vi "Send Barcode.vi"(8 "ErrorIn":errorcluster, 10 "Command":string, 11 "VISAIn":refnum<visa-resource-name>) -> (0 "ErrorOut":errorcluster, 2 "Data":string, 3 "VISAOut":refnum<visa-resource-name>)   [LabVIEW 2017, in "I28Drivers.lvlib"]
uses:
  I28Drivers.lvlib
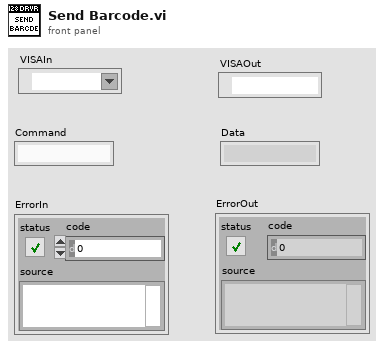
[diagram p1: front panel]
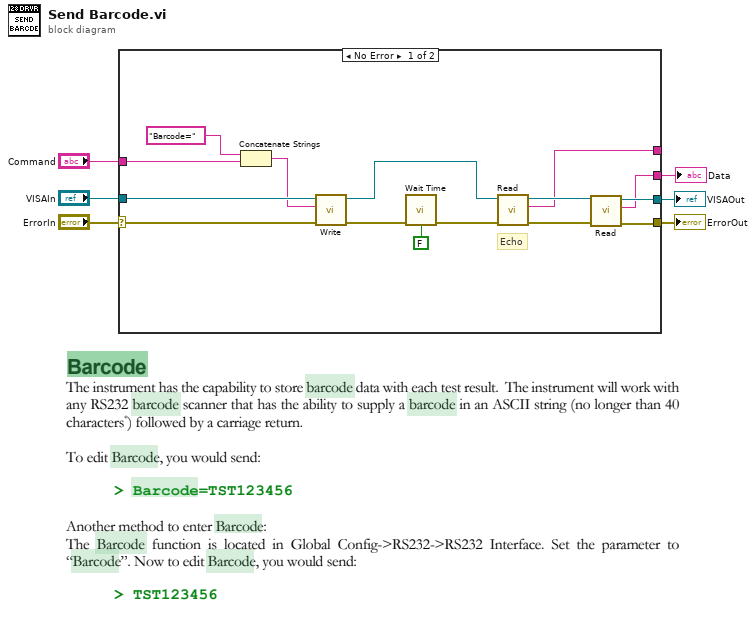
[diagram p0: block diagram]
diagram:
  n1 = case shown="No Error" "ErrorIn" {
    selector: "ErrorIn" -> [w21 w22]
    tunnel: "VISAIn" -> [w20 w23]
    tunnel: "Command" -> [w19 _]
    tunnel: [w16 w22] -> w3
    tunnel: [w15 w23] -> w2
    tunnel: [w14 _] -> w1
    tunnel: [w11 _] -> _
    frame No Error {
      # "Echo"
      n2 = Concatenate Strings("Barcode=" ("string"), w19) -> (w17:string)
      n3 = call "Write.vi"("ErrorIn"=w21, "Command"=w17, "VISAIn"=w20) -> ("ErrorOut"=w9:errorcluster, "VISAOut"=w10:refnum<visa-resource-name>)  [unwired: 7 in]
      n4 = call "Wait Time.vi"("error in"=w9, "Set Time"=FALSE) -> ("error out"=w8:errorcluster)  [unwired: 13 in]
      n5 = call "Read.vi"("ErrorIn"=w8, "VISAIn"=w10) -> ("ErrorOut"=w13:errorcluster, "Data"=w11:string, "VISAOut"=w12:refnum<visa-resource-name>)  [unwired: 7 in]
      n6 = call "Read.vi"("ErrorIn"=w13, "VISAIn"=w12) -> ("ErrorOut"=w16:errorcluster, "Data"=w14:string, "VISAOut"=w15:refnum<visa-resource-name>)  [unwired: 7 in]
    }
    frame Error {
    }
  }
  "ErrorOut" <- w3
  "VISAOut" <- w2
  "Data" <- w1
